vi "deltaCalculations.vi"() -> ()   [LabVIEW 2015]
uses:
  Global Distance.vi
  Global Angle.vi
panel:
  out "dy":dbl
  out "dz":dbl
  out "dis":dbl
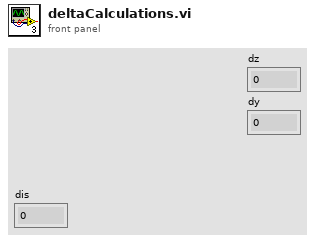
[diagram p1: front panel]
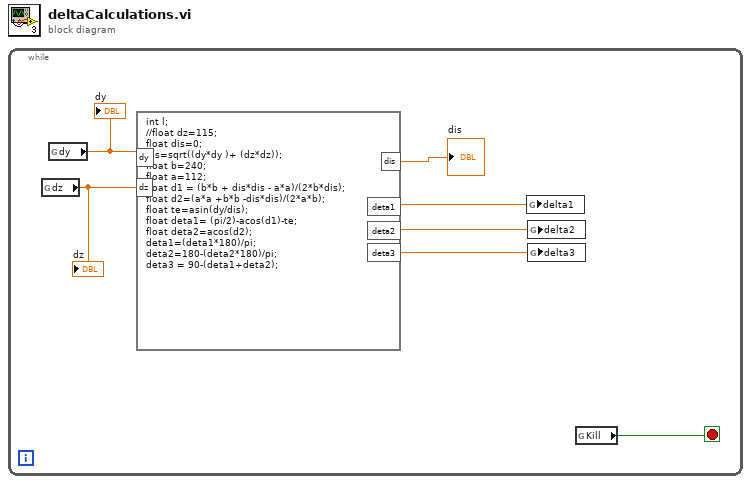
[diagram p0: block diagram]
diagram:
  n1 = while {
    stop <- w1 stop-if-true
    n2 = global read "Global Distance.vi" "dz"() -> (w3:dbl)
    "dz" <- w3
    n3 = global read "Global Distance.vi" "dy"() -> (w6:dbl)
    "dy" <- w6
    n4 = formula code="int l;\n//float dz=115;\nfloat dis=0;\ndis=sqrt((dy*dy )+ (dz*dz));\nfloat b=240;\nfloat a=112;\nfloat d1 = (b*b + dis*dis - a*a)/(2*b*dis);\nfloat d2=(a*a +b*b -dis*dis)/(2*a*b);\nfloat te=asin(dy/dis);\nfloat deta1= (pi/2)-acos(d1)-te;\nfloat deta2=acos(d2);\ndeta1=(deta1*180)/pi;\ndeta2=180-(deta2*180)/pi;\ndeta3 = 90-(deta1+deta2);"("dy"=w6, "dz"=w3) -> ("deta1"=w5:dbl, "deta2"=w4:dbl, "dis"=→"dis":dbl, "deta3"=w2:dbl)
    n5 = global write "Global Distance.vi" "delta1"(w5) -> ()
    n6 = global write "Global Distance.vi" "delta2"(w4) -> ()
    n7 = global write "Global Distance.vi" "delta3"(w2) -> ()
    n8 = global read "Global Angle.vi" "Kill"() -> (w1:bool)
  }
